vi "DblArray_Build Time List.vi"(4 "dt":dbl=1.0, 5 "Size":i32) -> (1 "Time Array":dbl[](array[numeric]))   [LabVIEW 2024, in "WavBuf.lvclass"]
uses:
  WavBuf/WavBuf.lvclass
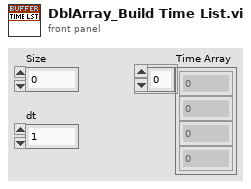
[diagram p1: front panel]
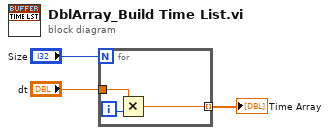
[diagram p0: block diagram]
diagram:
  n1 = for {
    N: "Size" -> [_]
    tunnel: "dt" -> [w5]
    tunnel: [w4] -> w1 mode=indexing
    i -> [w6]
    n2 = Multiply(x=w5, y=w6) -> (x*y=w4:dbl)
  }
  "Time Array" <- w1
